vi "Monitor Humidity.vi"(8 "error in (no error)":errorcluster, 10 "Address (0)":i32, 11 "VISA resource name":refnum<visa-resource-name>) -> (0 "error out":errorcluster, 1 "humidity setpoint":dbl, 2 "measured humidity":dbl, 3 "VISA resource name out":refnum<visa-resource-name>, 4 "lower limit alarm":dbl, 5 "upper limit alarm":dbl)   [LabVIEW 2016, in "Environment Chamber.lvlib" / "Climatic Chamber.lvlib"]
doc: "<b>Humidity setting monitor</B>\n\nMonitors information related to the humidity."
uses:
  Climatic Chamber.lvlib
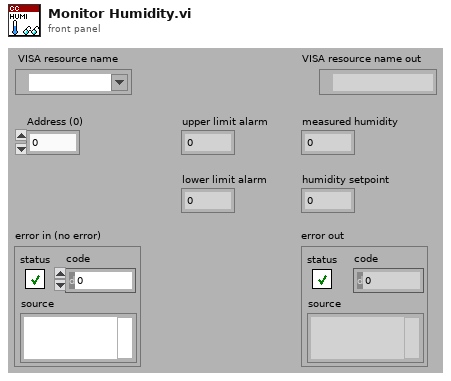
[diagram p1: front panel]
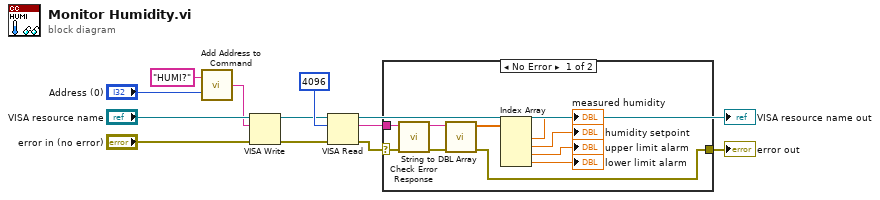
[diagram p0: block diagram]
diagram:
  n1 = call "Add Address to Command.vi"("Address (0)"="Address (0)", "Command"="HUMI?") -> ("Command OUT"=w4:string)
  n2 = VISA Write(VISA resource name="VISA resource name", write buffer=w4, error in (no error)="error in (no error)") -> (VISA resource name out=w9:refnum<visa-resource-name>, error out=w8:errorcluster)  [unwired: 1 out]
  n3 = VISA Read(VISA resource name=w9, byte count=u32 4096, error in (no error)=w8) -> (VISA resource name out=→"VISA resource name out":refnum<visa-resource-name>, read buffer=w2:string, error out=w3:errorcluster)  [unwired: 1 out]
  n4 = case shown="No Error" w3 {
    selector: w3 -> [w17 w23]
    tunnel: w2 -> [w18 _]
    tunnel: [w13 w23] -> w1
    frame No Error {
      n5 = call "Check Error Response.vi"("error in (no error)"=w17, "read String"=w18) -> ("error out"=w15:errorcluster, "String out"=w16:string)  [unwired: 7 in, 1 out]
      n6 = call "String to DBL Array.vi"("error in (no error)"=w15, "String received"=w16) -> ("error out"=w13:errorcluster, "Array Data"=w14:dbl[])  [unwired: 8 in]
      n7 = Index Array(array=w14) -> (element #1=→"measured humidity":dbl, element #2=→"humidity setpoint":dbl, element #3=→"upper limit alarm":dbl, element #4=→"lower limit alarm":dbl)  [unwired: 4 in]
    }
    frame Error {
    }
  }
  "error out" <- w1
